vi "Config Dual ARB.vi"(0 "VISA Resource Name":refnum<visa-resource-name>, 1 "Reconstruction Filter (1:2.5MHZ)":T1(ring)=enum."2.5 MHZ", 2 "ARB Reference (F:INT)":bool, 3 "Reference Freq (10.00000000)":dbl=10.0 format="%.8f", 5 "Select Waveform (T:ARBI)":bool=TRUE, 7 "File (ARB_DATA)":string="ARB_DATA", 9 "ARB Sample Clock (10.0)":dbl=10.0 format="%.8f", 11 "error in (no error)":errorcluster {"code" format="%.0x"}) -> (4 "VISA Resource Name Out":refnum<visa-resource-name>, 15 "error out":errorcluster {"code" format="%.0x"})   [LabVIEW 2014, in "Agilent ESG Series.lvlib"]
doc: "This VI is used to configure PDC pattern data.\n\nThis VI is valid only on instruments with the UND option or on Agilent E4438C instrument with option 001/601 or 002/602."
uses:
  Agilent ESG Series.lvlib
panel:
  # "ARBI:"
  # "SEQ:"
  # "EXT"
  # "INT"
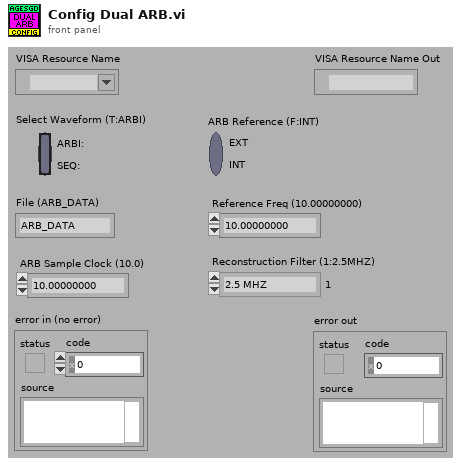
[diagram p1: front panel]
types:
  T1 = enum16{"250 KHZ", "2.5 MHZ", "8.0 MHZ", "THROUGH"}
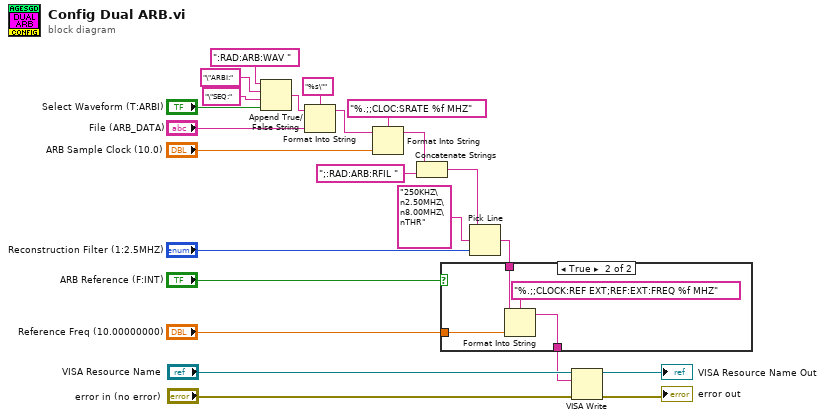
[diagram p0: block diagram]
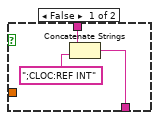
[diagram p2: hidden frame]
diagram:
  n1 = Append True/False String(1:"Select Waveform (T:ARBI)", 2:"\"SEQ:" ("false string"), 3:"\"ARBI:" ("true string"), 4:":RAD:ARB:WAV " ("string (\"\")")) -> (0:w3:string)
  n2 = Format Into String(format string="%s\"", initial string=w3, "File (ARB_DATA)") -> (resulting string=w17:string)  [unwired: 1 in, 1 out]
  n3 = Format Into String(format string="%.;;CLOC:SRATE %f MHZ", initial string=w17, "ARB Sample Clock (10.0)") -> (resulting string=w16:string)  [unwired: 1 in, 1 out]
  n4 = Concatenate Strings(w16, ";:RAD:ARB:RFIL " ("string (\"\")")) -> (w12:string)
  n5 = Pick Line(string ("")=w12, multi-line string="250KHZ\n2.50MHZ\n8.00MHZ\nTHR", line index="Reconstruction Filter (1:2.5MHZ)") -> (output string=w13:string)
  n6 = case shown="True" "ARB Reference (F:INT)" {
    tunnel: w13 -> [w26 w30]
    tunnel: [w24 w27] -> w8
    tunnel: "Reference Freq (10.00000000)" -> [_ w28]
    frame False {
      n7 = Concatenate Strings(w26, ";CLOC:REF INT") -> (w24:string)
    }
    frame True {
      n8 = Format Into String(format string="%.;;CLOCK:REF EXT;REF:EXT:FREQ %f MHZ", initial string=w30, w28) -> (resulting string=w27:string)  [unwired: 1 in, 1 out]
    }
  }
  n9 = VISA Write(VISA resource name="VISA Resource Name", write buffer=w8, error in (no error)="error in (no error)") -> (VISA resource name out=→"VISA Resource Name Out":refnum<visa-resource-name>, error out=→"error out":errorcluster)  [unwired: 1 out]
